vi "read_excel_values.vi"() -> ()   [LabVIEW 2024]
uses:
  <vilib>/addons/_office/excel.llb/Excel Get Data ([dbl]).vi
  <vilib>/addons/_office/excel.llb/Excel Get Data ([str]).vi
  <vilib>/addons/_office/excel.llb/Excel Get Data (i32).vi
  <vilib>/Utility/NIReport.llb/NI_report.lvclass
  <vilib>/Utility/NIReport.llb/Excel/NI_Excel.lvclass
  <vilib>/addons/_office/NI_ReportGenerationToolkit.lvlib
panel:
  out "Sheet 3 Data":i32
  out "Sheet 2 Data":string[][](array[string])
  out "Sheet 1 Data":dbl[][](array[numeric]) format="%.2f"
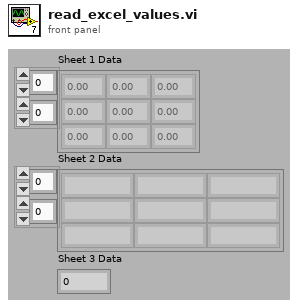
[diagram p1: front panel]
types:
  T1 = enum16{"Standard Report", "HTML", "Word", "Excel"}
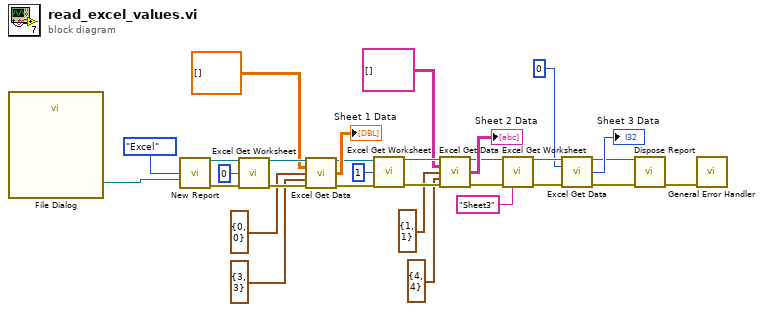
[diagram p0: block diagram]
diagram:
  n1 = call "File Dialog"() -> ("selected path"=w10:path)  [unwired: 7 in, 8 out]
  n2 = call <vilib>:"New Report.vi"("report type"=T1."Excel", "template (empty)"=w10) -> ("report out"=w30:refnum<class "NI_report.lvclass">, "error out"=w21:errorcluster)  [unwired: 4 in, 8 out]
  n3 = call <vilib>:"Excel Get Worksheet.vi"("report in"=w30, "worksheet index (0)"=0, "error in (no error)"=w21) -> ("report out"=w29:refnum<class "NI_report.lvclass">, "error out"=w20:errorcluster)  [unwired: 11 out]
  n4 = call-poly <vilib>:"Excel Get Data.vi"("report in"=w29, "data type"=dbl[][] [], "start (-1, -1)"=cluster{"row":i32, "column":i32} {"row"=0, "column"=0}, "end (-1, -1)"=cluster{"row":i32, "column":i32} {"row"=3, "column"=3}, "error in (no error)"=w20) -> ("report out"=w24:refnum<class "NI_report.lvclass">, "data"=→"Sheet 1 Data":dbl[][], "error out"=w16:errorcluster)  [unwired: 8 out]
  n5 = call <vilib>:"Excel Get Worksheet.vi"("report in"=w24, "worksheet index (0)"=1, "error in (no error)"=w16) -> ("report out"=w22:refnum<class "NI_report.lvclass">, "error out"=w15:errorcluster)  [unwired: 11 out]
  n6 = call-poly <vilib>:"Excel Get Data.vi"("report in"=w22, "data type"=string[][] [], "start (-1, -1)"=cluster{"row":i32, "column":i32} {"row"=1, "column"=1}, "end (-1, -1)"=cluster{"row":i32, "column":i32} {"row"=4, "column"=4}, "error in (no error)"=w15) -> ("report out"=w7:refnum<class "NI_report.lvclass">, "data"=→"Sheet 2 Data":string[][], "error out"=w5:errorcluster)  [unwired: 8 out]
  n7 = call <vilib>:"Excel Get Worksheet.vi"("report in"=w7, "error in (no error)"=w5, "name (\"\")"="Sheet3" ("name (\"\")")) -> ("report out"=w8:refnum<class "NI_report.lvclass">, "error out"=w9:errorcluster)  [unwired: 1 in, 10 out]
  n8 = call-poly <vilib>:"Excel Get Data.vi"("report in"=w8, "data type"=0, "error in (no error)"=w9) -> ("report out"=w1:refnum<class "NI_report.lvclass">, "data"=→"Sheet 3 Data":i32, "error out"=w6:errorcluster)  [unwired: 1 in, 9 out]
  n9 = call-dynamic "Dispose Report.vi"("report in"=w1, "error in (no error)"=w6) -> ("error out"=w17:errorcluster)  [unwired: 3 in, 10 out]
  n10 = call <vilib>:"General Error Handler.vi"("error in (no error)"=w17) -> ()  [unwired: 3 in, 12 out]
